vi "addFrames.vi"() -> ()   [LabVIEW 2015]
uses:
  GlobalPath.vi
  GlobalData.vi
  GlobalVi.vi
panel:
  out "PanelName":string
  in  "EXT 6":string
  in  "EXT 5":string
  in  "DONE ALL?":bool
  in  "INT 4":string
  in  "INT 3":string
  in  "INT 2":string
  in  "ptfe 2":bool caption="Position the 6 external frames using the 12 PTFE pins"
  in  "visual 4":bool caption="Position the 4 internal frames"
  in  "Save the IDs in the database?":bool
  in  "Fill database with all 10 frame IDs?\nTo do so go to the database, select the Frame tab, choose the correct frame ID and press \"check_db\"\nThen click on \"Add/Update Entry\"":bool
  in  "INT 1":string
  in  "EXT 4":string
  in  "EXT 3":string
  in  "EXT 2":string
  in  "EXT 1":string
  # "1. Add frame on table/stiffback"
  # "3. Adding the frames to the database"
  # "Scan the ID of each of the 10 frames and associate them with the panel"
  # "2. Frame ID recording"
  # "Fill each box with the correct IDs and press SAVE"
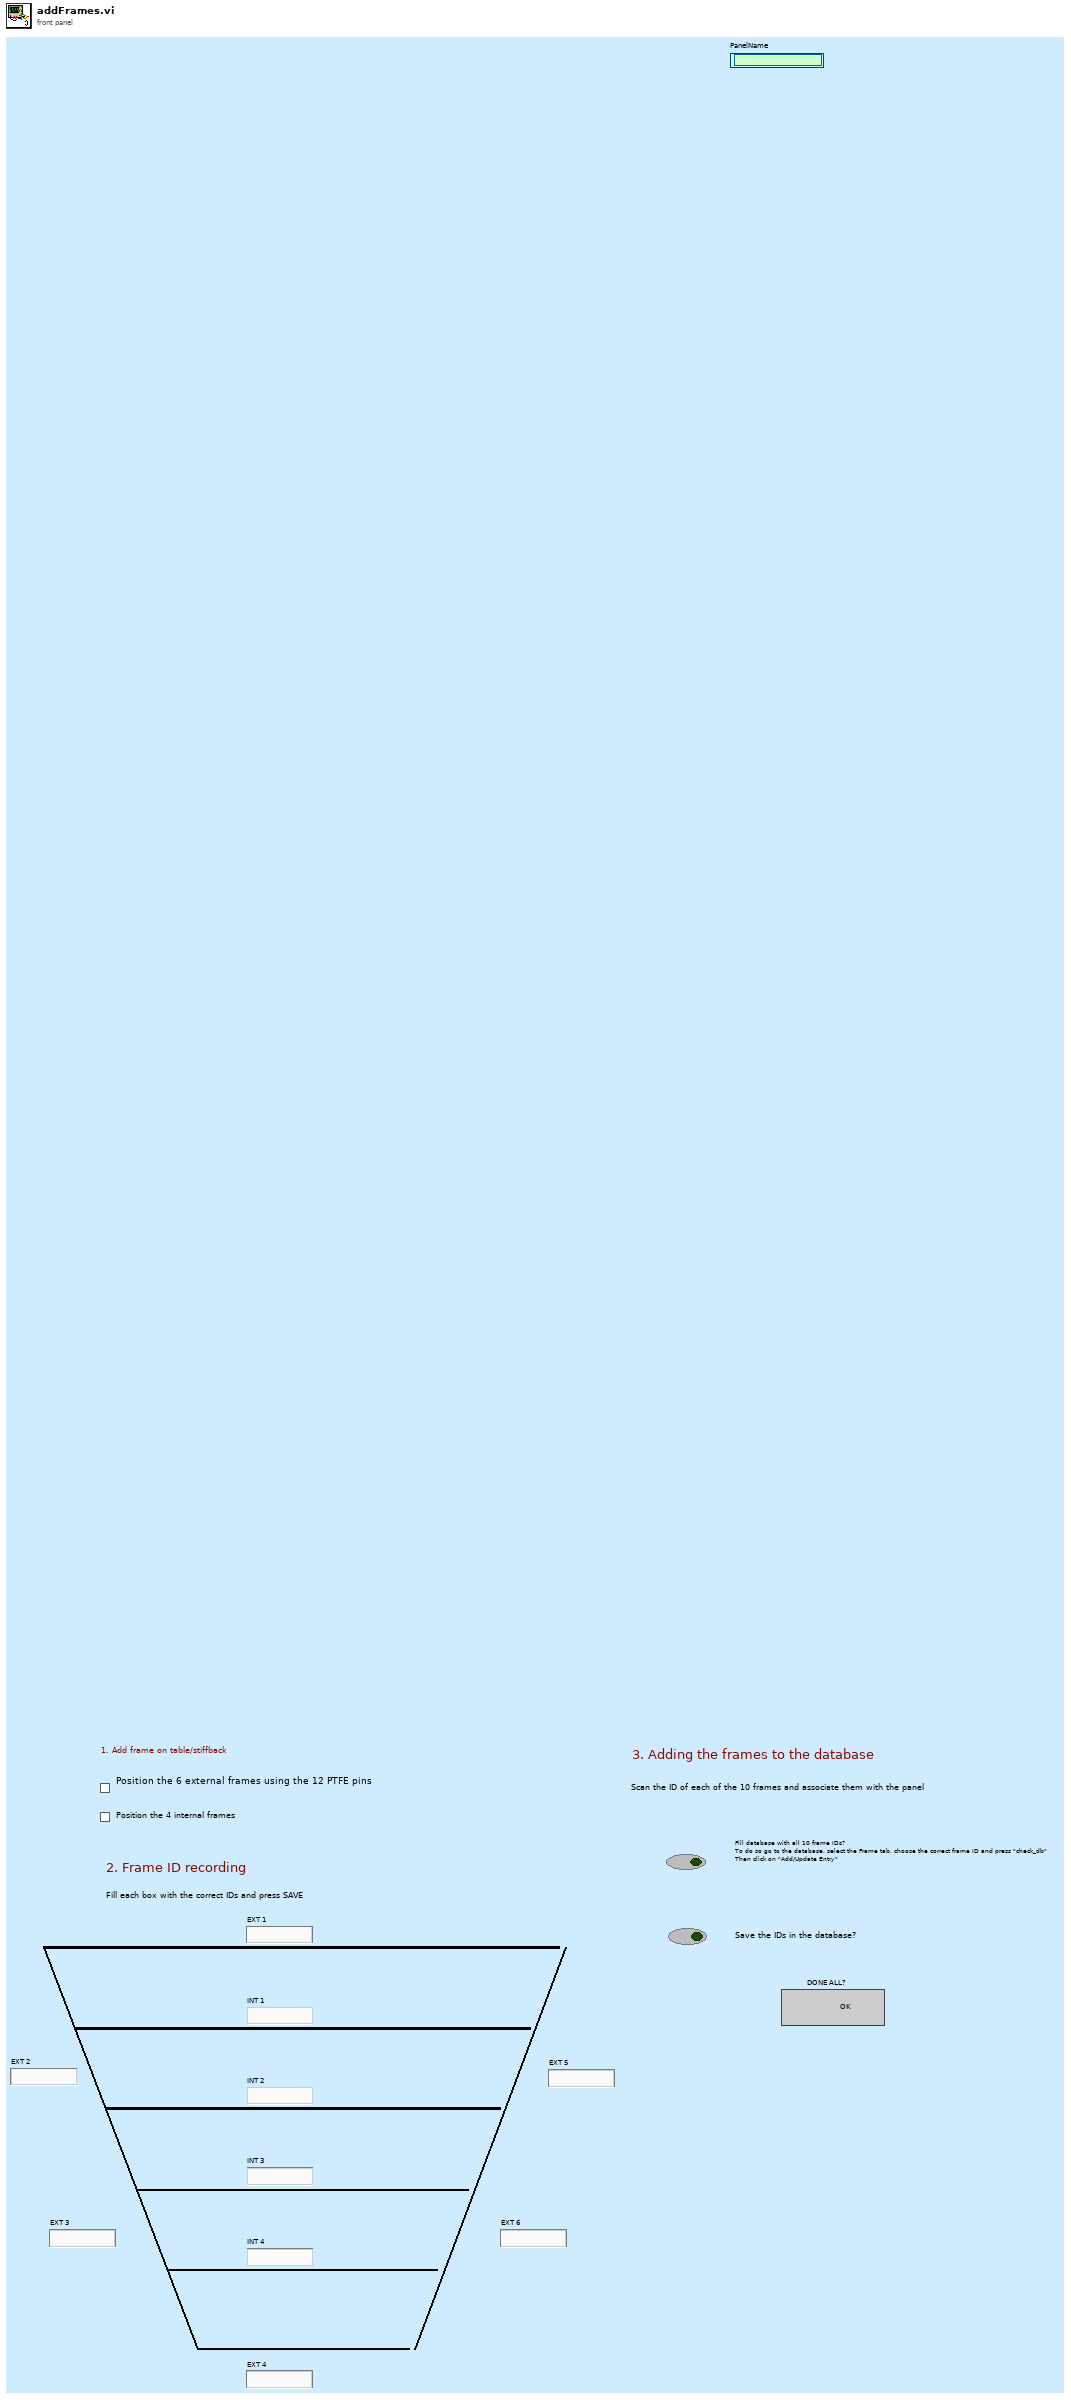
[diagram p1: front panel]
types:
  T1 = enum16{"open", "replace", "create", "open or create", "replace or create", "replace or create with confirmation"}
  T2 = enum32{"Bad", "Idle", "Run top level", "Running"}
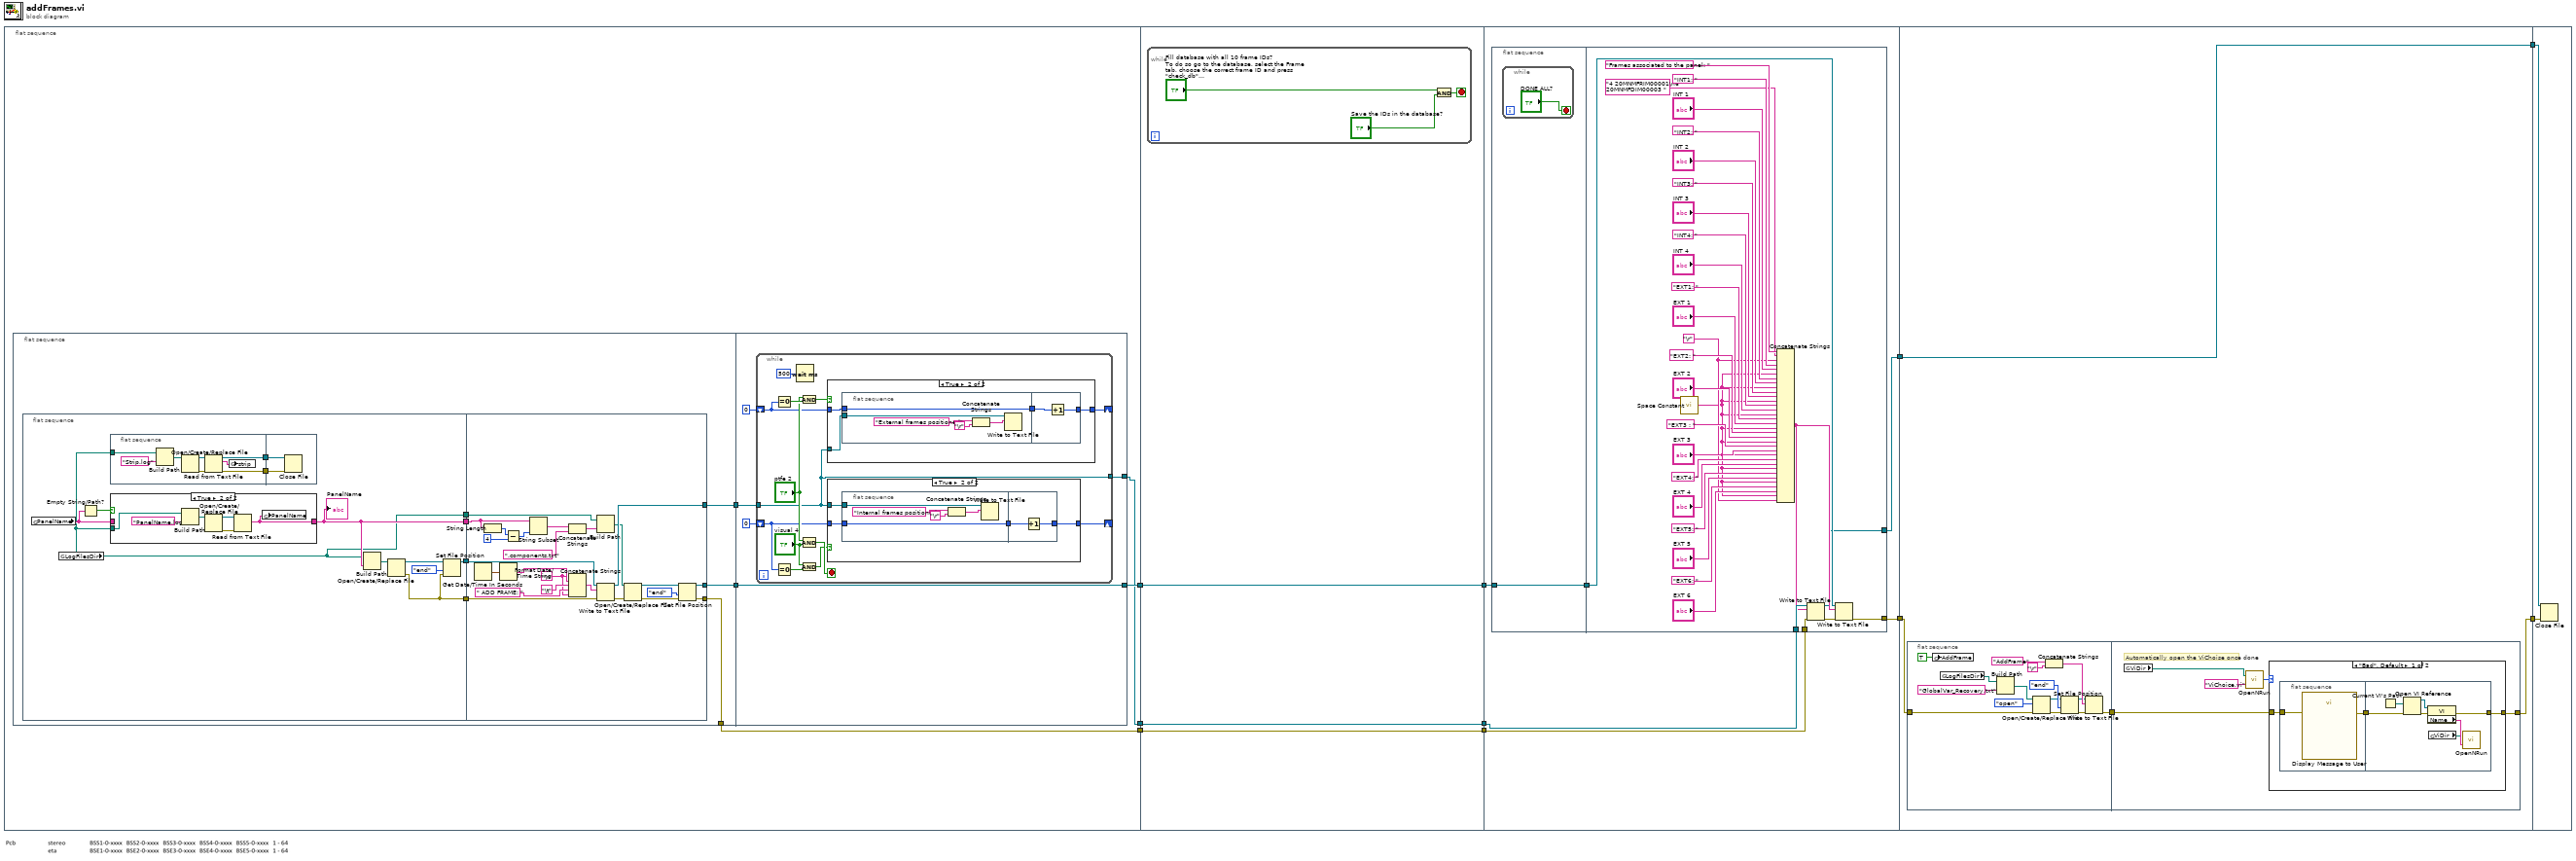
[diagram p0: block diagram]
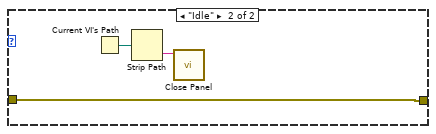
[diagram p5: hidden frame]
diagram:
  n1 = flat-sequence {
    tunnel: [w11] -> w10
    tunnel: [w14] -> w9
    tunnel: [w12] -> w1
    tunnel: w10 -> [w119]
    tunnel: [w119] -> w4
    tunnel: w9 -> [w118]
    tunnel: [w118] -> w3
    tunnel: [w117] -> w2
    tunnel: w1 -> [w117]
    tunnel: w4 -> [w127]
    tunnel: [w124] -> w7
    tunnel: w3 -> [w128]
    tunnel: [w123] -> w6
    tunnel: w2 -> [w126]
    tunnel: [w164] -> w8
    tunnel: w7 -> [w162]
    tunnel: w6 -> [w165]
    tunnel: [w165] -> w5
    tunnel: w8 -> [w201]
    tunnel: w5 -> [w202]
    frame #0 {
      n2 = flat-sequence {
        tunnel: [w21] -> w15
        tunnel: [w20] -> w14
        tunnel: [w16] -> w13
        tunnel: w15 -> [w79]
        tunnel: w13 -> [w76]
        tunnel: [w76] -> w12
        tunnel: [w75] -> w11
        frame #0 {
          n3 = flat-sequence {
            tunnel: [w30] -> w22
            tunnel: [w32] -> w19
            tunnel: [w25] -> w18
            tunnel: [w23] -> w17
            tunnel: w22 -> [w70]
            tunnel: [w69] -> w21
            tunnel: [w53] -> w20
            tunnel: w19 -> [w55]
            tunnel: w18 -> [w51]
            tunnel: w17 -> [w60]
            tunnel: [w52] -> w16
            frame #0 {
              n4 = global read "GlobalData.vi" "PanelName"() -> (w29:string)
              n5 = global read "GlobalPath.vi" "LogFilesDir"() -> (w23:path)
              n6 = Empty String/Path?(string/path=w29) -> (empty?=w28:bool)
              n7 = flat-sequence {
                tunnel: w23 -> [w41]
                tunnel: [w35] -> w27
                tunnel: [w34] -> w26
                tunnel: w27 -> [w43]
                tunnel: w26 -> [w42]
                frame #0 {
                  n8 = Build Path(base path=w41, name or relative path="Strip.log") -> (appended path=w40:path)
                  n9 = Open/Create/Replace File(file path (use dialog)=w40) -> (refnum out=w37:refnum<file>, error out=w38:errorcluster)  [unwired: 5 in, 1 out]
                  n10 = Read from Text File(file (use dialog)=w37, error in=w38) -> (refnum out=w34:refnum<file>, text=w36:string, error out=w35:errorcluster)  [unwired: 2 in, 1 out]
                  n11 = global write "GlobalData.vi" "strip"(w36) -> ()
                }
                frame #1 {
                  n12 = Close File(refnum=w42, error in=w43) -> ()  [unwired: 2 out]
                }
              }
              n13 = case shown="True" w28 {
                tunnel: w23 -> [_ w50]
                tunnel: [w44 w45] -> w25
                tunnel: w29 -> [w44 _]
                frame False {
                }
                frame True {
                  n14 = Build Path(base path=w50, name or relative path="PanelName.log") -> (appended path=w49:path)
                  n15 = Open/Create/Replace File(file path (use dialog)=w49) -> (refnum out=w46:refnum<file>, error out=w47:errorcluster)  [unwired: 5 in, 1 out]
                  n16 = Read from Text File(file (use dialog)=w46, error in=w47) -> (text=w45:string)  [unwired: 2 in, 3 out]
                  n17 = global write "GlobalData.vi" "PanelName"(w45) -> ()
                }
              }
              "PanelName" <- w25
              n18 = Build Path(base path=w23, name or relative path=w25) -> (appended path=w24:path)
              n19 = Open/Create/Replace File(file path (use dialog)=w24) -> (refnum out=w31:refnum<file>, error out=w32:errorcluster)  [unwired: 5 in, 1 out]
              n20 = Set File Position(refnum=w31, from (0:start)=enum16{"start", "end", "current"}."end", error in=w32) -> (refnum out=w30:refnum<file>)  [unwired: 1 in, 1 out]
            }
            frame #1 {
              w67 = "\r"
              n21 = Get Date/Time In Seconds() -> (seconds since 1Jan1904=w68:timestamp)
              n22 = String Length(string=w51) -> (length=w64:i32)
              n23 = Format Date/Time String(seconds (now)=w68) -> (date/time string=w72:string)  [unwired: 2 in]
              n24 = Subtract(x=w64, y=4) -> (x-y=w63:i32)
              n25 = String Subset(string=w51, length (rest)=w63) -> (substring=w62:string)  [unwired: 1 in]
              n26 = Concatenate Strings(w62, ".components.txt") -> (w66:string)
              n27 = Concatenate Strings(w67, w72, "\t", " ADD FRAME: ", w67) -> (w71:string)
              n28 = Build Path(base path=w60, name or relative path=w66) -> (appended path=w56:path)
              n29 = Write to Text File(file (use dialog)=w70, text=w71, error in=w55) -> (refnum out=w69:refnum<file>, error out=w54:errorcluster)  [unwired: 1 in, 1 out]
              n30 = Open/Create/Replace File(file path (use dialog)=w56, error in=w54) -> (refnum out=w58:refnum<file>, error out=w59:errorcluster)  [unwired: 4 in, 1 out]
              n31 = Set File Position(refnum=w58, from (0:start)=enum16{"start", "end", "current"}."end", error in=w59) -> (refnum out=w52:refnum<file>, error out=w53:errorcluster)  [unwired: 1 in]
            }
          }
        }
        frame #1 {
          n32 = while {
            tunnel: w79 -> [w80]
            shift-right: [w81] -> _
            shift-left: 0 -> [w87]
            shift-right: [w82] -> _
            shift-left: 0 -> [w83]
            tunnel: [w80] -> w75
            stop <- w92 stop-if-true
            n33 = Equal To 0?(x=w87) -> (x = 0?=w90:bool)
            n34 = Equal To 0?(x=w83) -> (x = 0?=w86:bool)
            n35 = Wait (ms)(milliseconds to wait=u32 500) -> ()  [unwired: 1 out]
            n36 = And(x="ptfe 2", y=w90) -> (x .and. y?=w89:bool)
            n37 = And(x="visual 4", y=w86) -> (x .and. y?=w85:bool)
            n38 = Compound Arithmetic op=AND("ptfe 2", "visual 4") -> (w92:bool)
            n39 = case shown="True" w89 {
              tunnel: w80 -> [_ w109]
              tunnel: w87 -> [w105 w107]
              tunnel: [w105 w106] -> w81
              frame False {
              }
              frame True {
                n40 = flat-sequence {
                  tunnel: w109 -> [w111]
                  tunnel: [w110] -> w108
                  tunnel: w107 -> [w110]
                  tunnel: w108 -> [w116]
                  tunnel: [w115] -> w106
                  frame #0 {
                    n41 = Concatenate Strings("External frames positioned", "\r") -> (w114:string)
                    n42 = Write to Text File(file (use dialog)=w111, text=w114) -> ()  [unwired: 2 in, 3 out]
                  }
                  frame #1 {
                    n43 = Increment(x=w116) -> (x+1=w115:i32)
                  }
                }
              }
            }
            n44 = case shown="True" w85 {
              tunnel: w80 -> [_ w97]
              tunnel: w83 -> [w93 w95]
              tunnel: [w93 w94] -> w82
              frame False {
              }
              frame True {
                n45 = flat-sequence {
                  tunnel: w97 -> [w99]
                  tunnel: [w98] -> w96
                  tunnel: w95 -> [w98]
                  tunnel: w96 -> [w104]
                  tunnel: [w103] -> w94
                  frame #0 {
                    n46 = Concatenate Strings("Internal frames positioned", "\r") -> (w102:string)
                    n47 = Write to Text File(file (use dialog)=w99, text=w102) -> ()  [unwired: 2 in, 3 out]
                  }
                  frame #1 {
                    n48 = Increment(x=w104) -> (x+1=w103:i32)
                  }
                }
              }
            }
          }
        }
      }
    }
    frame #1 {
      n49 = while {
        stop <- w120 stop-if-true
        n50 = And(x="Fill database with all 10 frame IDs?\nTo do so go to the database, select the Frame tab, choose the correct frame ID and press \"check_db\"\nThen click on \"Add/Update Entry\"", y="Save the IDs in the database?") -> (x .and. y?=w120:bool)
      }
    }
    frame #2 {
      n51 = flat-sequence {
        tunnel: w126 -> [w129]
        tunnel: [w129] -> w125
        tunnel: w128 -> [w160]
        tunnel: w127 -> [w159]
        tunnel: w125 -> [w137]
        tunnel: [w131] -> w124
        tunnel: [w132] -> w123
        frame #0 {
          n52 = while {
            stop <- "DONE ALL?" stop-if-true
          }
        }
        frame #1 {
          w139 = "\r"
          n53 = call <vilib>:"Space Constant.vi"() -> ("String"=w138:string)
          n54 = Concatenate Strings("Frames associated to the panel: ", "4 20MNMFRIM00001\n6 20MNMFDIM00003 ", w139, "INT1: ", "INT 1", w138, "INT2: ", "INT 2", w138, "INT3: ", "INT 3", w138, "INT4: ", "INT 4", w138, "EXT1: ", "EXT 1", w138, "EXT2: ", "EXT 2", w138, "EXT3 : ", "EXT 3", w138, "EXT4: ", "EXT 4", w138, "EXT5: ", "EXT 5", w138, "EXT6: ", "EXT 6", w138, w139) -> (w136:string)
          n55 = Write to Text File(file (use dialog)=w159, text=w136, error in=w160) -> (refnum out=w132:refnum<file>, error out=w135:errorcluster)  [unwired: 1 in, 1 out]
          n56 = Write to Text File(file (use dialog)=w137, text=w136, error in=w135) -> (error out=w131:errorcluster)  [unwired: 1 in, 2 out]
        }
      }
    }
    frame #3 {
      n57 = flat-sequence {
        tunnel: [w168] -> w163
        tunnel: w162 -> [w169]
        tunnel: [w181] -> w164
        tunnel: w163 -> [w182]
        frame #0 {
          n58 = global write "GlobalVi.vi" "AddFrame"(TRUE) -> ()
          n59 = global read "GlobalPath.vi" "LogFilesDir"() -> (w166:path)
          n60 = Build Path(base path=w166, name or relative path="GlobalVar_Recovery.txt") -> (appended path=w178:path)
          n61 = Open/Create/Replace File(file path (use dialog)=w178, error in=w169, operation (0:open)=T1."open") -> (refnum out=w174:refnum<file>, error out=w175:errorcluster)  [unwired: 3 in, 1 out]
          n62 = Concatenate Strings("AddFrame", "\r") -> (w173:string)
          n63 = Set File Position(refnum=w174, from (0:start)=enum16{"start", "end", "current"}."end", error in=w175) -> (refnum out=w171:refnum<file>, error out=w170:errorcluster)  [unwired: 1 in]
          n64 = Write to Text File(file (use dialog)=w171, text=w173, error in=w170) -> (error out=w168:errorcluster)  [unwired: 1 in, 2 out]
        }
        frame #1 {
          # "Automatically open the ViChoise once done"
          n65 = global read "GlobalPath.vi" "ViDir"() -> (w185:path)
          n66 = call "OpenNRun.vi"("VI name"="ViChoice.vi", "ViDirPath"=w185) -> ("Execution:State"=w184:T2)
          n67 = case shown="\"Bad\", Default" w184 {
            tunnel: [w186 w198] -> w181
            tunnel: w182 -> [w187 w198]
            frame "Bad", Default {
              n68 = flat-sequence {
                tunnel: w187 -> [w190]
                tunnel: [w189] -> w188
                tunnel: w188 -> [w194]
                tunnel: [w191] -> w186
                frame #0 {
                  n69 = call "Display Message to User"("error in (no error)"=w190) -> ("error out"=w189:errorcluster)  [unwired: 9 in, 1 out]
                }
                frame #1 {
                  n70 = Current VI's Path() -> (path=w192:path)
                  n71 = Open VI Reference(vi path=w192, error in (no error)=w194) -> (vi reference=w197:refnum<vi>, error out=w196:errorcluster)  [unwired: 4 in]
                  n72 = property class="VI"(reference=w197, error in=w196) -> (error out=w191:errorcluster, "Name"=w195:string)  [unwired: 1 out]
                  n73 = global read "GlobalPath.vi" "ViDir"() -> (w193:path)
                  n74 = call "OpenNRun.vi"("VI name"=w195, "ViDirPath"=w193) -> ()  [unwired: 1 out]
                }
              }
            }
            frame "Idle" {
              n75 = Current VI's Path() -> (path=w199:path)
              n76 = Strip Path(path=w199) -> (name=w200:string)  [unwired: 1 out]
              n77 = call <vilib>:"Close Panel.vi"("VI name"=w200) -> ()  [unwired: 10 in, 1 out]
            }
          }
        }
      }
    }
    frame #4 {
      n78 = Close File(refnum=w202, error in=w201) -> ()  [unwired: 2 out]
    }
  }
